vi "GetText.vi"(8 "error in":errorcluster, 11 "DIO Engine in":refnum<class "Digital IO Engine.lvclass">) -> (0 "error out":errorcluster, 1 "additional text":string, 2 "text":string, 3 "DIO Engine out":refnum<class "Digital IO Engine.lvclass">, 4 "glyph":string)   [LabVIEW 2025, in "Digital IO.lvlib" / "Digital IO Engine.lvclass"]
doc: "Copyright 2017 National Instruments Corporation\n\nLicensed under the Apache License, Version 2.0 (the \"License\"); you may not use this file except in compliance with the License. You may obtain a copy of the License at http://www.apache.org/licenses/LICENSE-2.0\nUnless required by applicable law or agreed to in writing, software distributed under the License is distributed on an \"AS IS\" BASIS, WITHOUT WARRANTIES OR CONDITIONS OF ANY KIND, either express or implied. See the License for the specific language governing permissions and limitations under the License."
uses:
  Digital IO Engine.lvclass
  Digital IO Engine.lvclass/Digital IO Engine.ctl
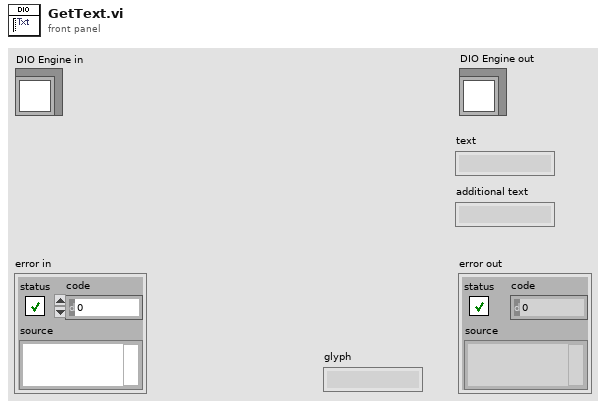
[diagram p1: front panel]
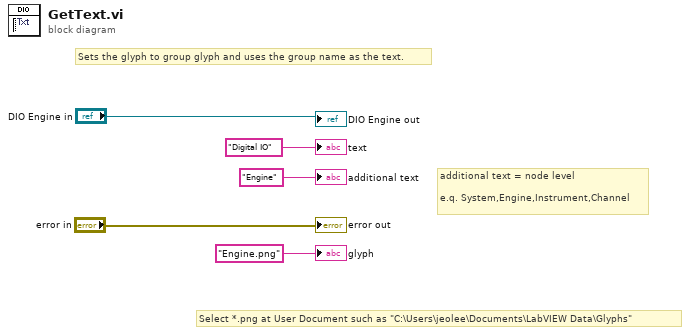
[diagram p0: block diagram]
diagram:
  # "Select *.png at User Document such as \"C:\\Users\\jeolee\\Documents\\LabVIEW Data\\Glyphs\""
  # "additional text = node level\n\ne.q. System,Engine,Instrument,Channel"
  # "Sets the glyph to group glyph and uses the group name as the text."
  "error out" <- "error in"
  "DIO Engine out" <- "DIO Engine in"
  "text" <- "Digital IO" ("text")
  "additional text" <- "Engine" ("text")
  "glyph" <- "Engine.png" ("glyph")
